vi "frequency_sweep.vi"() -> ()   [LabVIEW 2017]
uses:
  controls/State.ctl
  controls/Data.ctl
  <vilib>/Utility/error.llb/DialogType.ctl
  <vilib>/DAQmx/write.llb/DAQmx Write (Analog DBL 1Chan 1Samp).vi
  <vilib>/DAQmx/create/channels.llb/DAQmx Create Channel (AO-Voltage-Basic).vi
  <vilib>/DAQmx/miscellaneous.llb/DAQmx Fill In Error Info.vi
  <instrlib>/niVNA/niVNA.llb/niVNA Fetch Sweep Measurement (DBL).vi
panel:
  in  "Reference H Field On/Off":bool
  out "DAQ channel Out":tag="DAQ_6363/ao1"
  in  "Averaging Points":i32=4 min=1 max=3201 step=1
  in  "DAQ channel In":tag="DAQ_6363/ao1"
  in  "Exit Button":bool
  in  "IF Bandwidth":dbl(ring)=1000.0 items=["10 Hz"=10.0, "30 Hz"=30.0, "100 Hz"=100.0, "300 Hz"=300.0, "1 KHz"=1000.0, "3 KHz"=3000.0, "10 KHz"=10000.0, "30 KHz"=30000.0]
  in  "Reference H Field (Oe)":dbl=5500.0 min=-6000.0 max=6000.0
  in  "H Field (Oe)":dbl=1000.0 min=-6000.0 max=6000.0
  in  "Save Button":bool
  out "Status":string="Shutting down...Sweeping field to zero..."
  out "Cursor":cluster{"x":dbl, "y":dbl} {"x" format="%.2f"; "y" format="%.5f"}
  out "VNA Name Out":refnum<k15>="VNA_5630"
  out "Error Out":errorcluster
  in  "Error In (no error)":errorcluster
  in  "Format":i32(ring)=1 items=["Log Magnitude (dB)"=0, "Lin Magnitude"=1, "Phase (deg)"=2, "VSWR"=3, "Group Delay"=6]
  out "SpectrumGraph":cluster{"Field":dbl[], "Signal":dbl[]}(graph)
  in  "S-parameter":i32(ring)=1 caption="Measurement" items=["S11", "S21"]
  in  "Start Button":bool
  in  "Stop Button":bool
  in  "Output Power (dBm)":dbl=1.0 min=-25.0 max=5.0 step=0.5
  in  "Number of Points":i32=1000 min=1 max=3201 step=1
  in  "Stop frequency (GHz)":dbl=6.0 caption="Stop H Field (Oe)" min=0.01 max=6.0 format="%#_6f"
  in  "Start frequency (GHz)":dbl=1.0 min=0.01 max=6.0 format="%#_6f"
  in  "VNA Name In":refnum<k15>="VNA_5630"
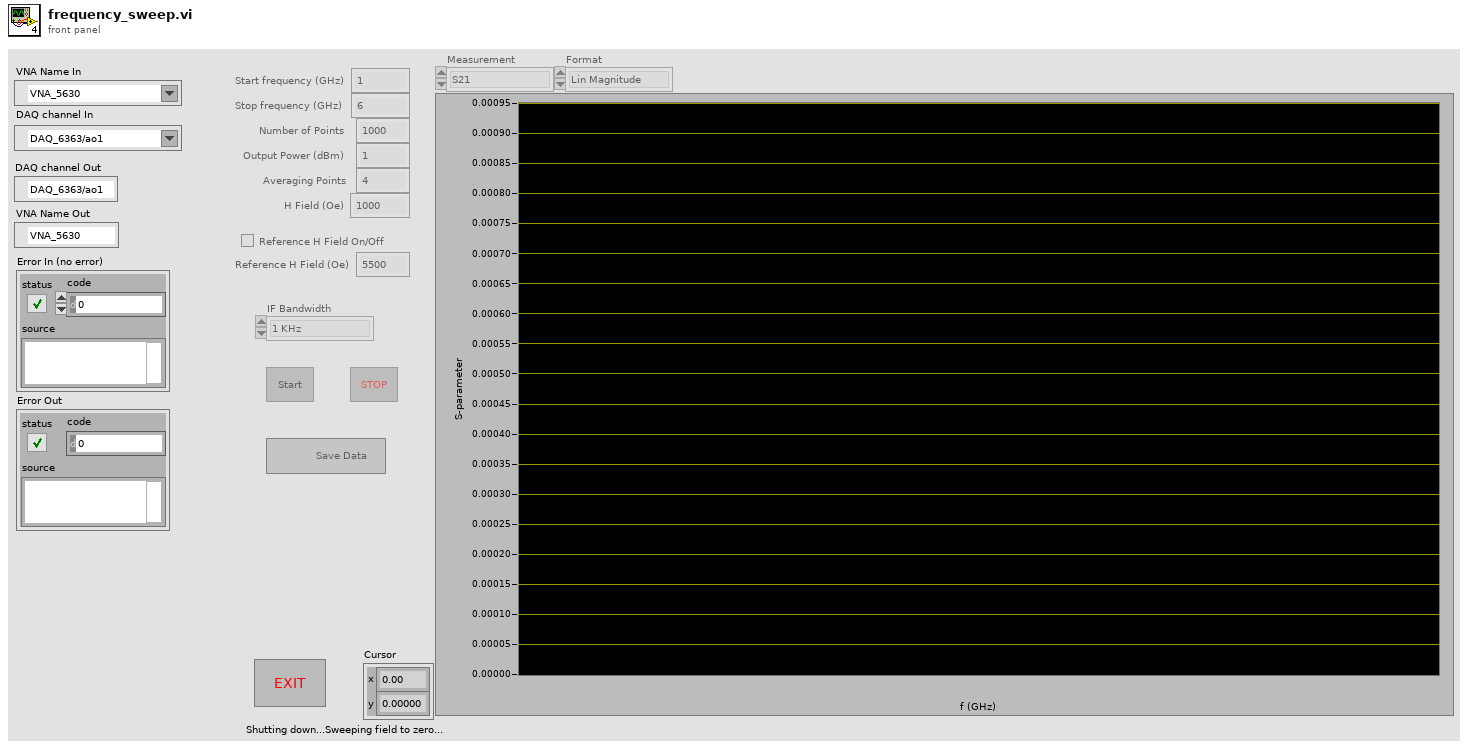
[diagram p1: front panel]
types:
  T1 = typedef "Data.ctl" = cluster{"Frequency":dbl[], "Signal":dbl[], "Ref signal":dbl[]}
  T2 = typedef "State.ctl" = enum16{"Init", "Idle", "Configuring", "Sweeping to ref", "Measuring ref", "Sweeping to H", "Measuring H", "Sweeping down", "Shutdown"}
  T3 = typedef "DialogType.ctl" = u16
  T4 = typedef "LVPoint32TypeDef.ctl" = cluster{"Horizontal":i32, "Vertical":i32}
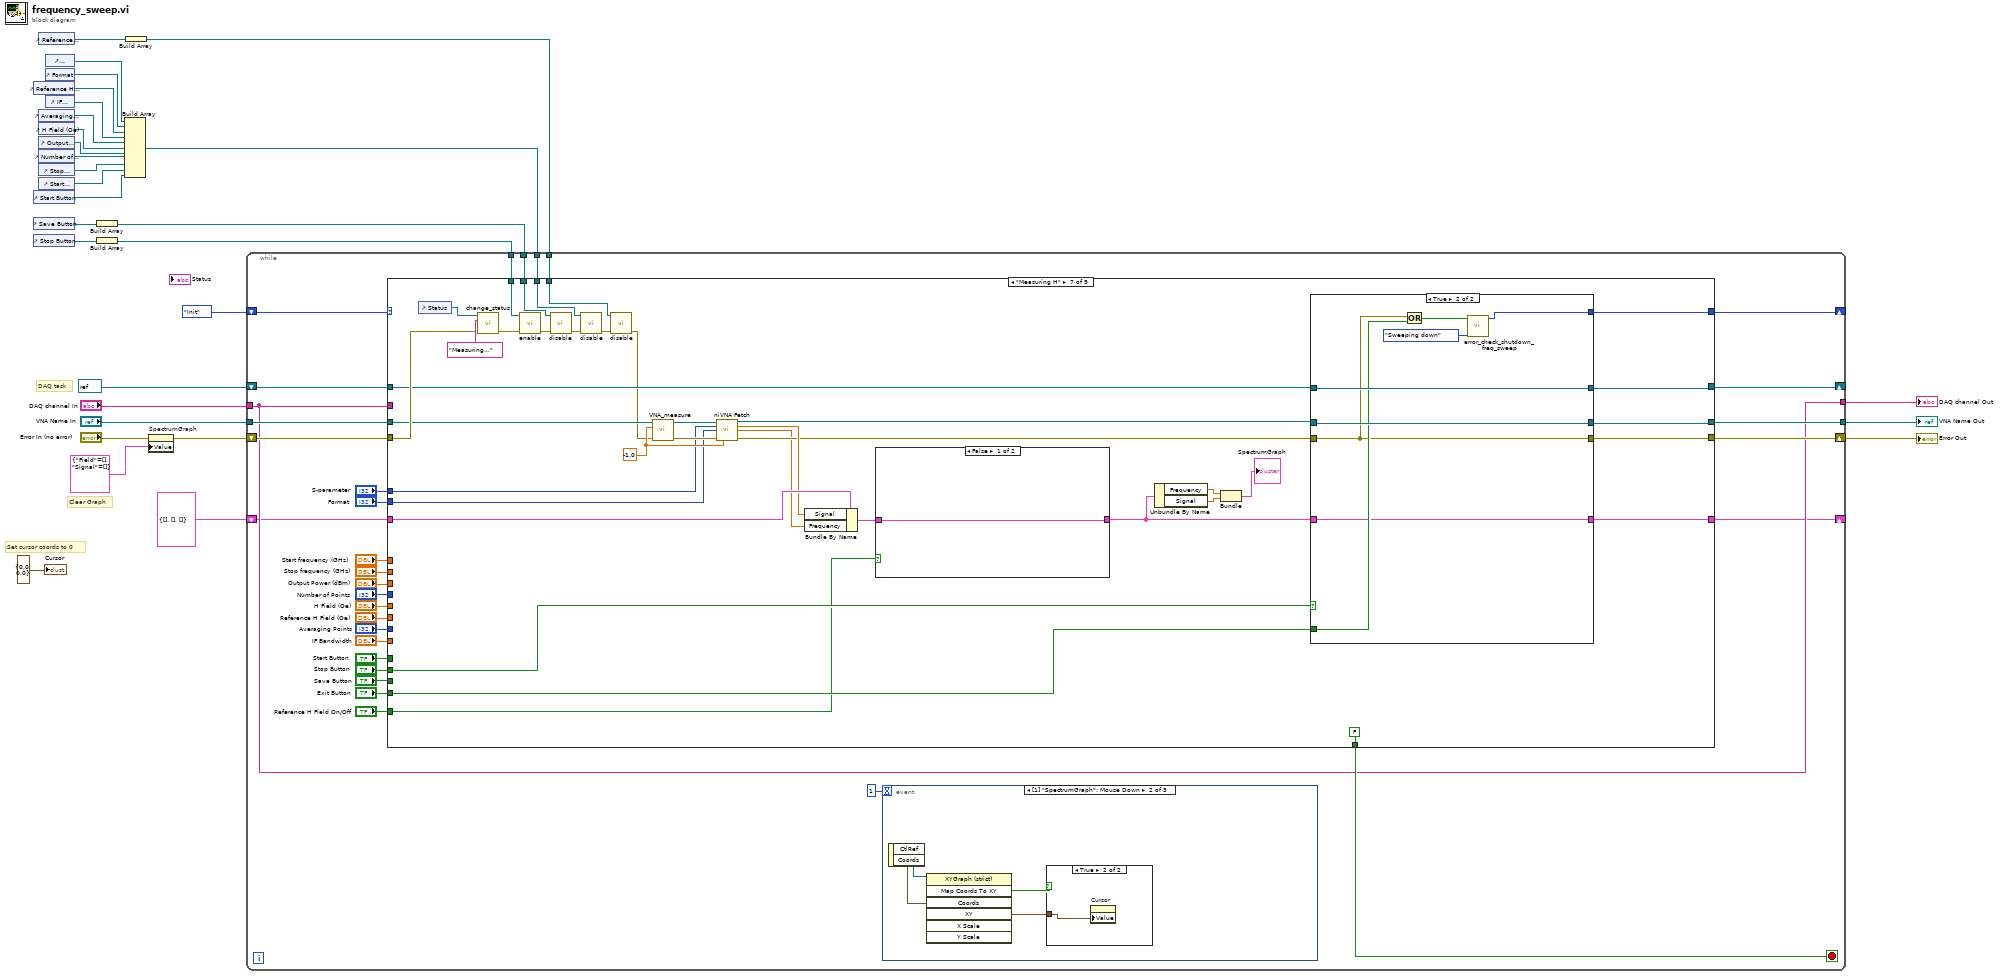
[diagram p0: block diagram]
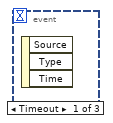
[diagram p2: hidden frame]
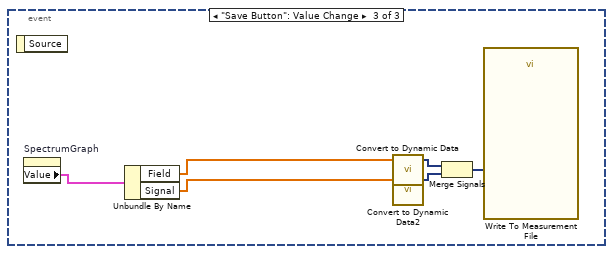
[diagram p4: hidden frame]
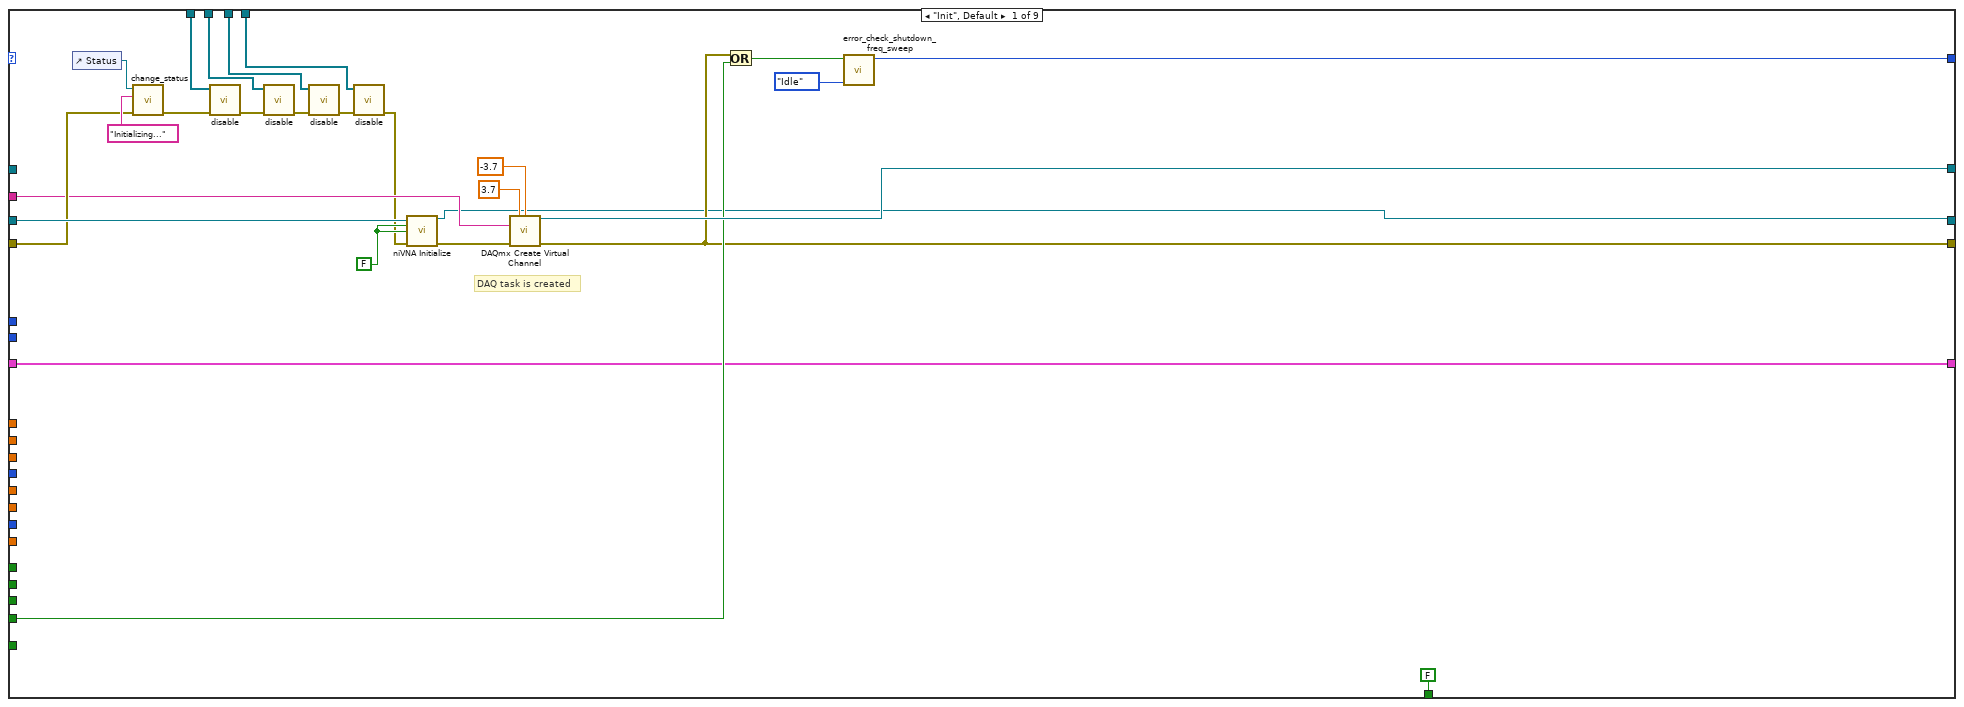
[diagram p5: hidden frame]
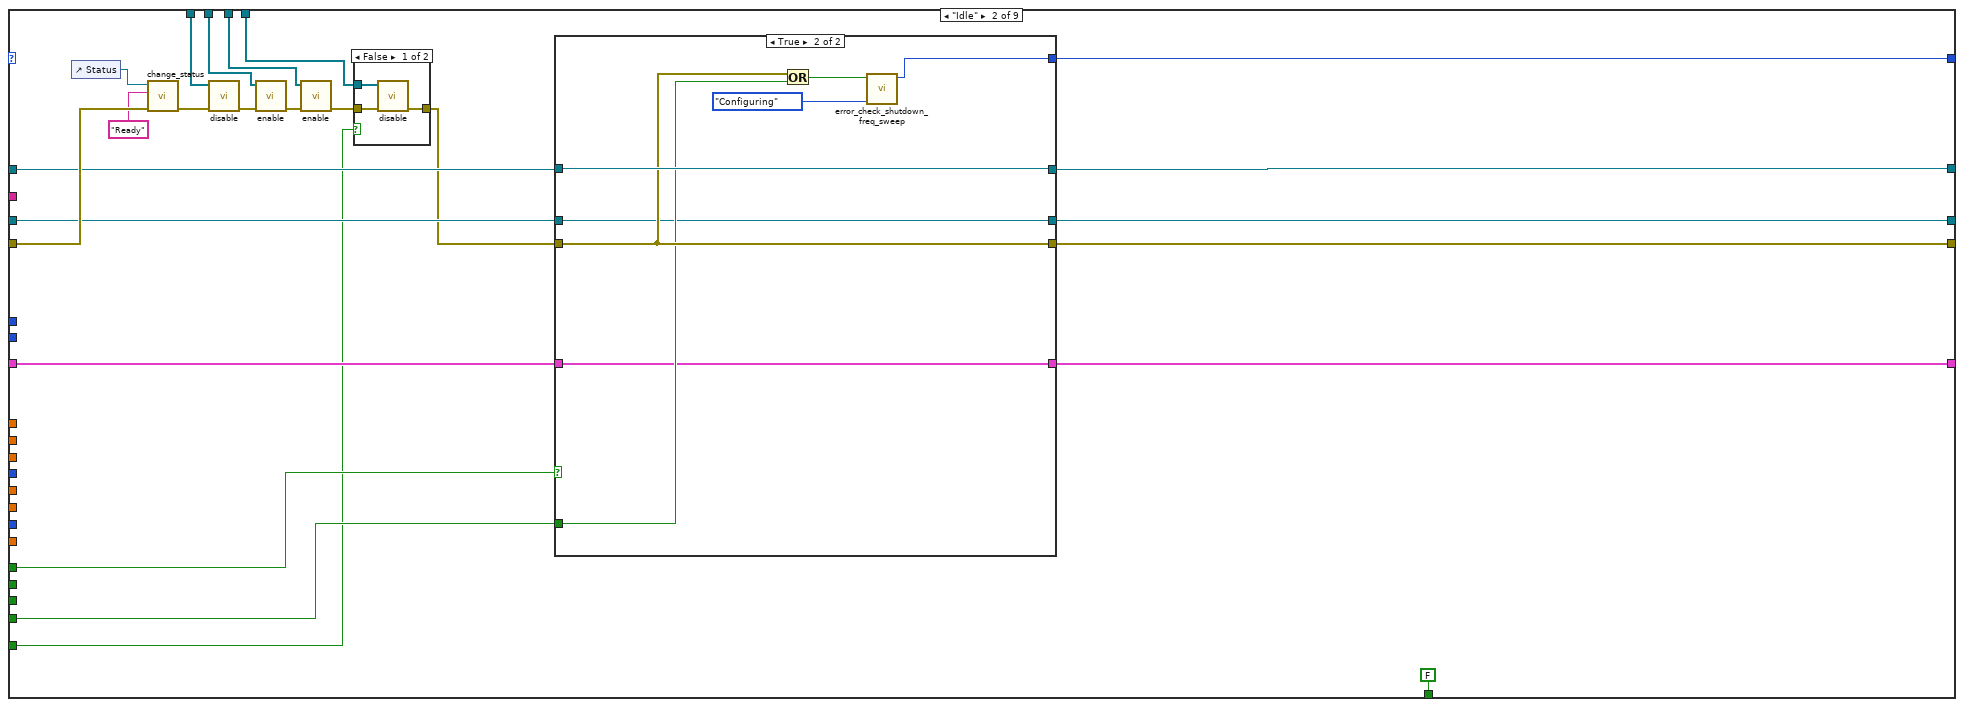
[diagram p6: hidden frame]
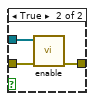
[diagram p7: hidden frame]
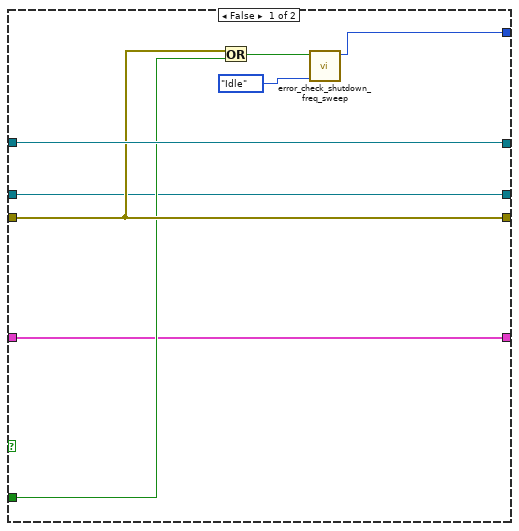
[diagram p8: hidden frame]
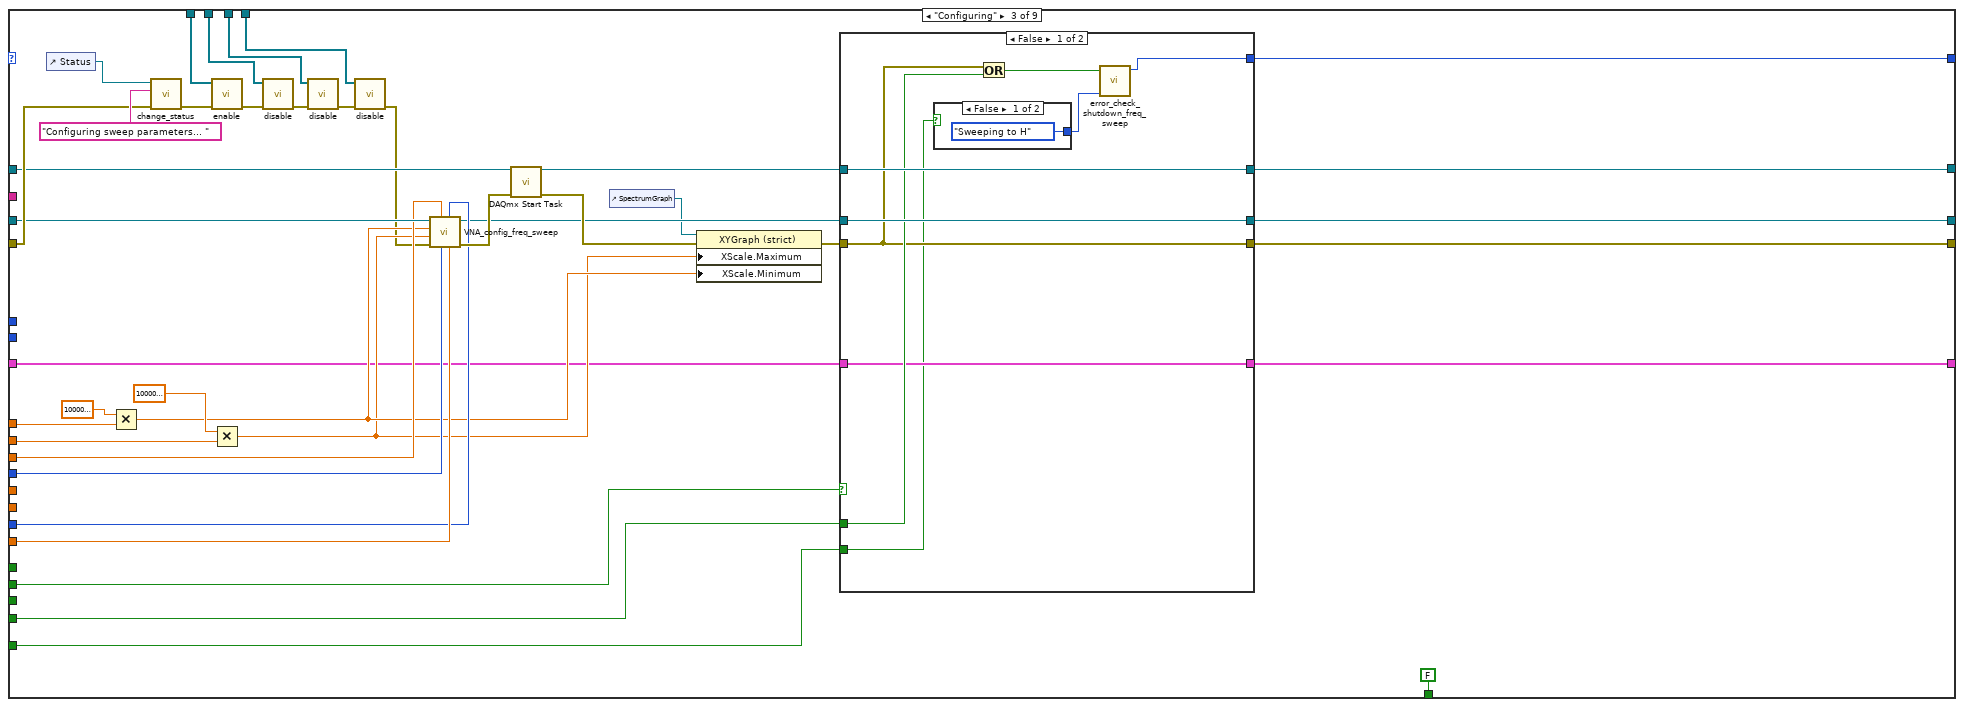
[diagram p9: hidden frame]
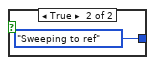
[diagram p10: hidden frame]
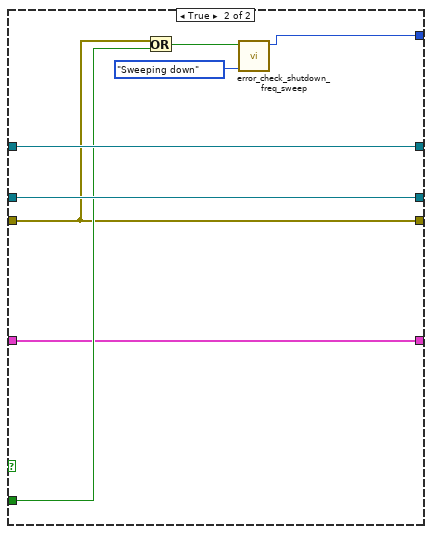
[diagram p11: hidden frame]
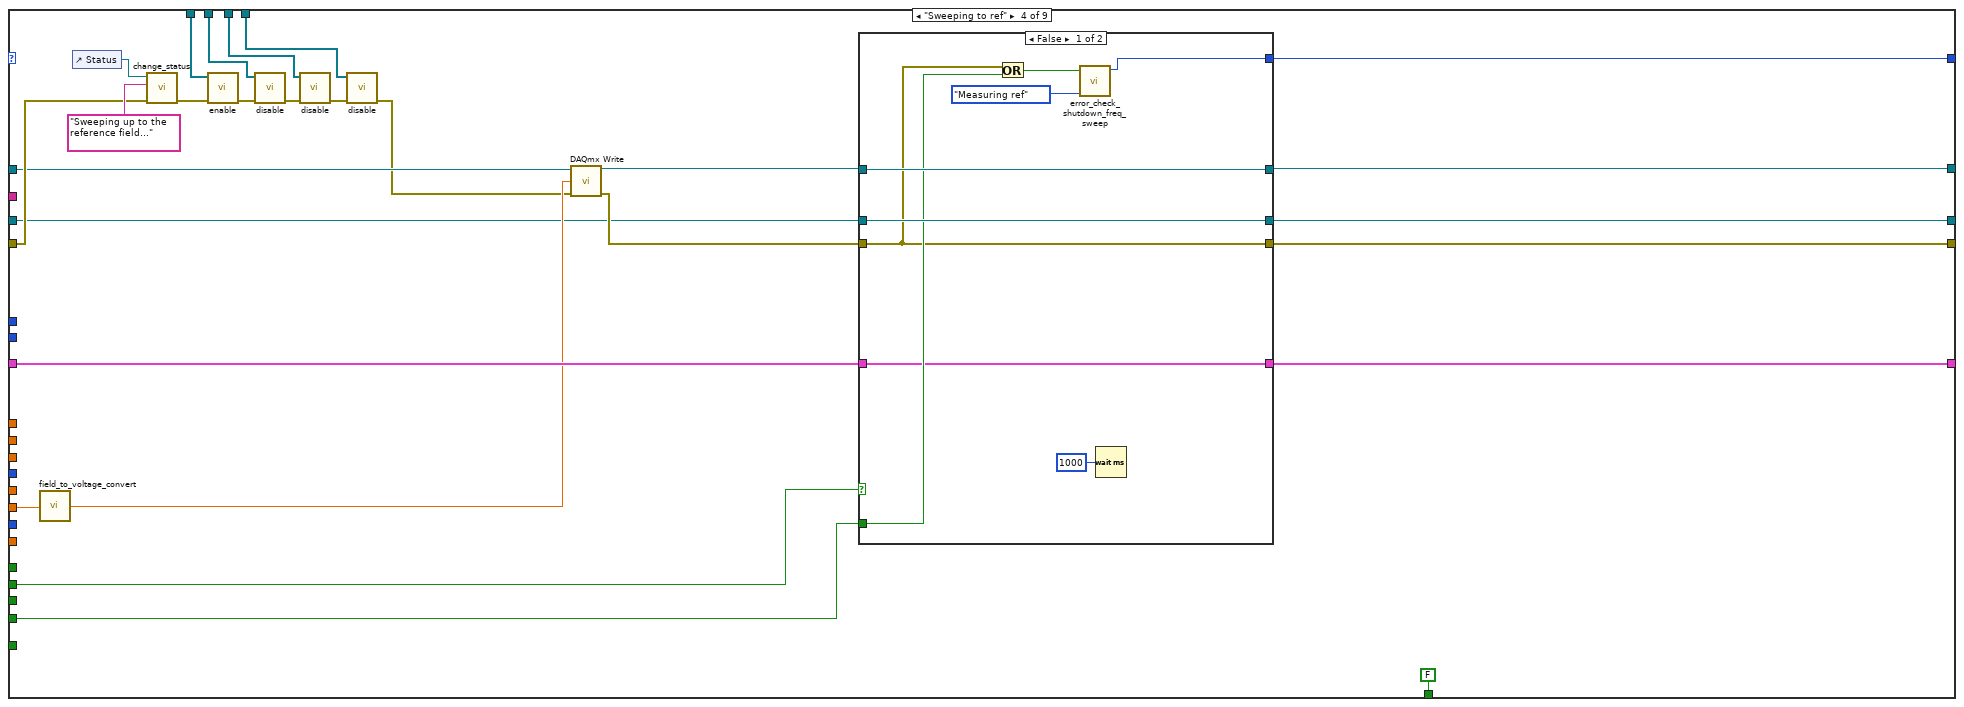
[diagram p12: hidden frame]
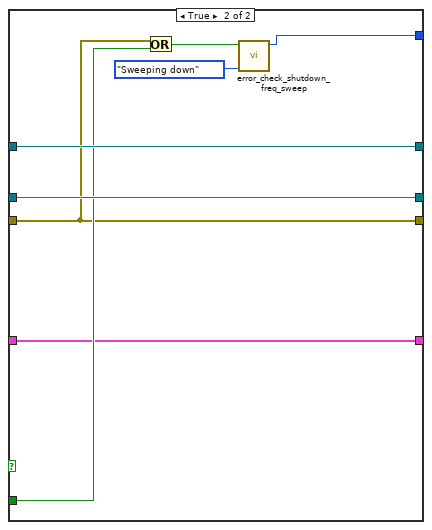
[diagram p13: hidden frame]
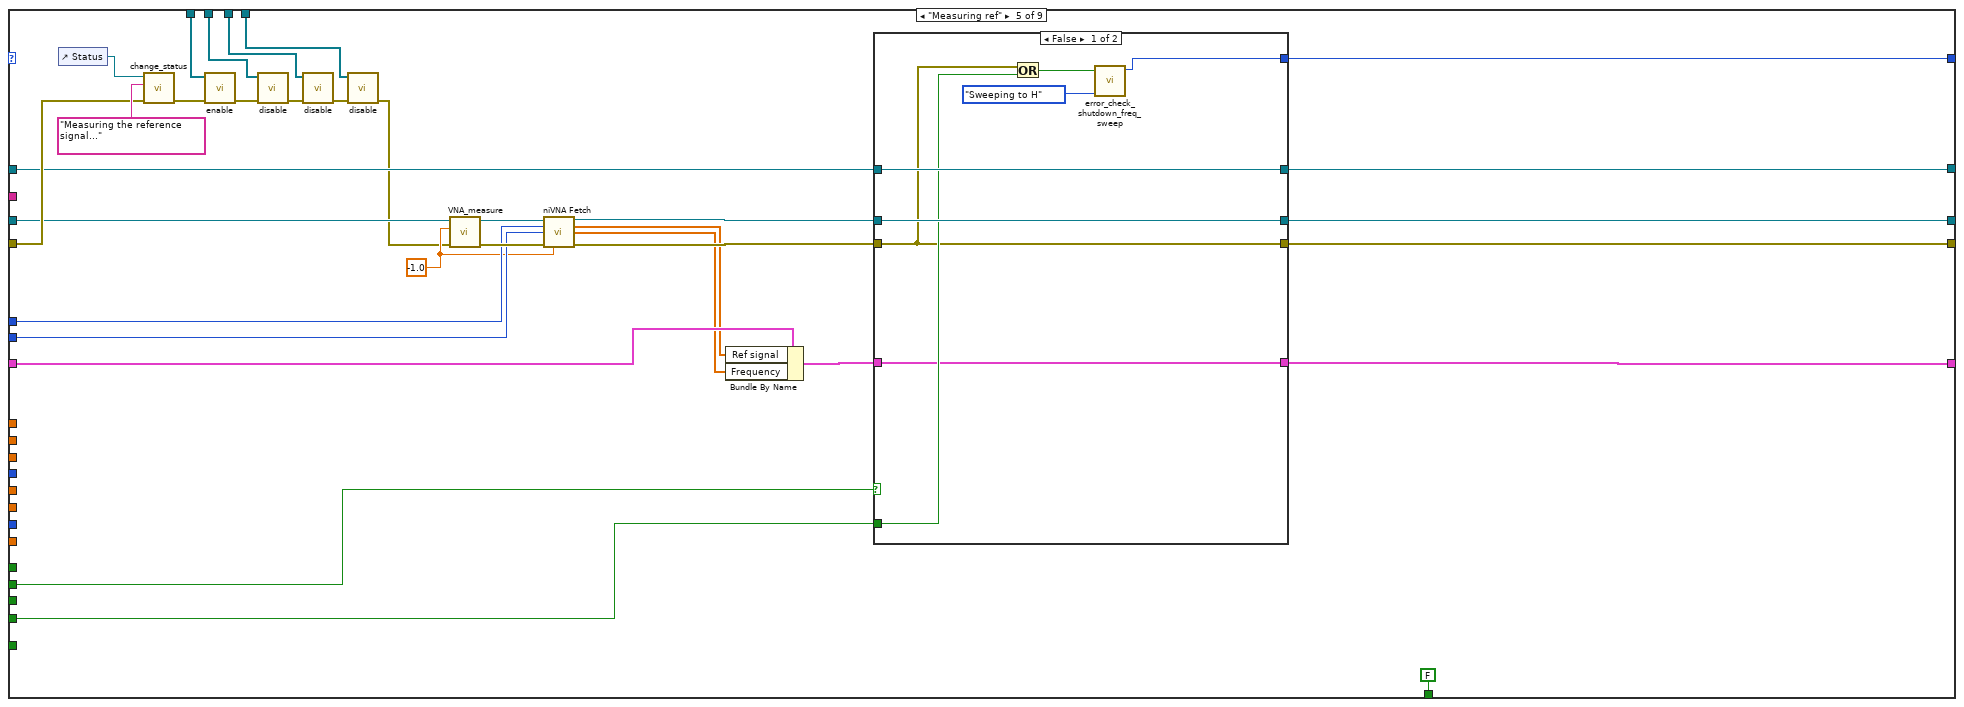
[diagram p14: hidden frame]
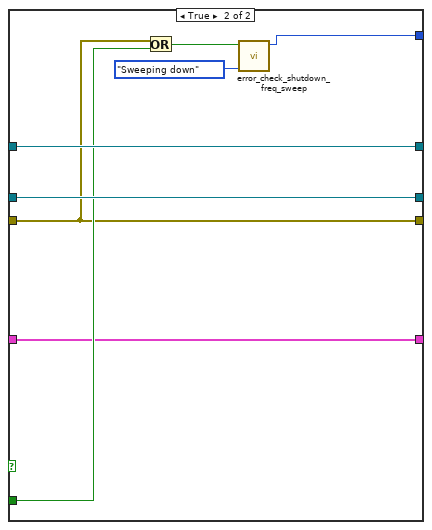
[diagram p15: hidden frame]
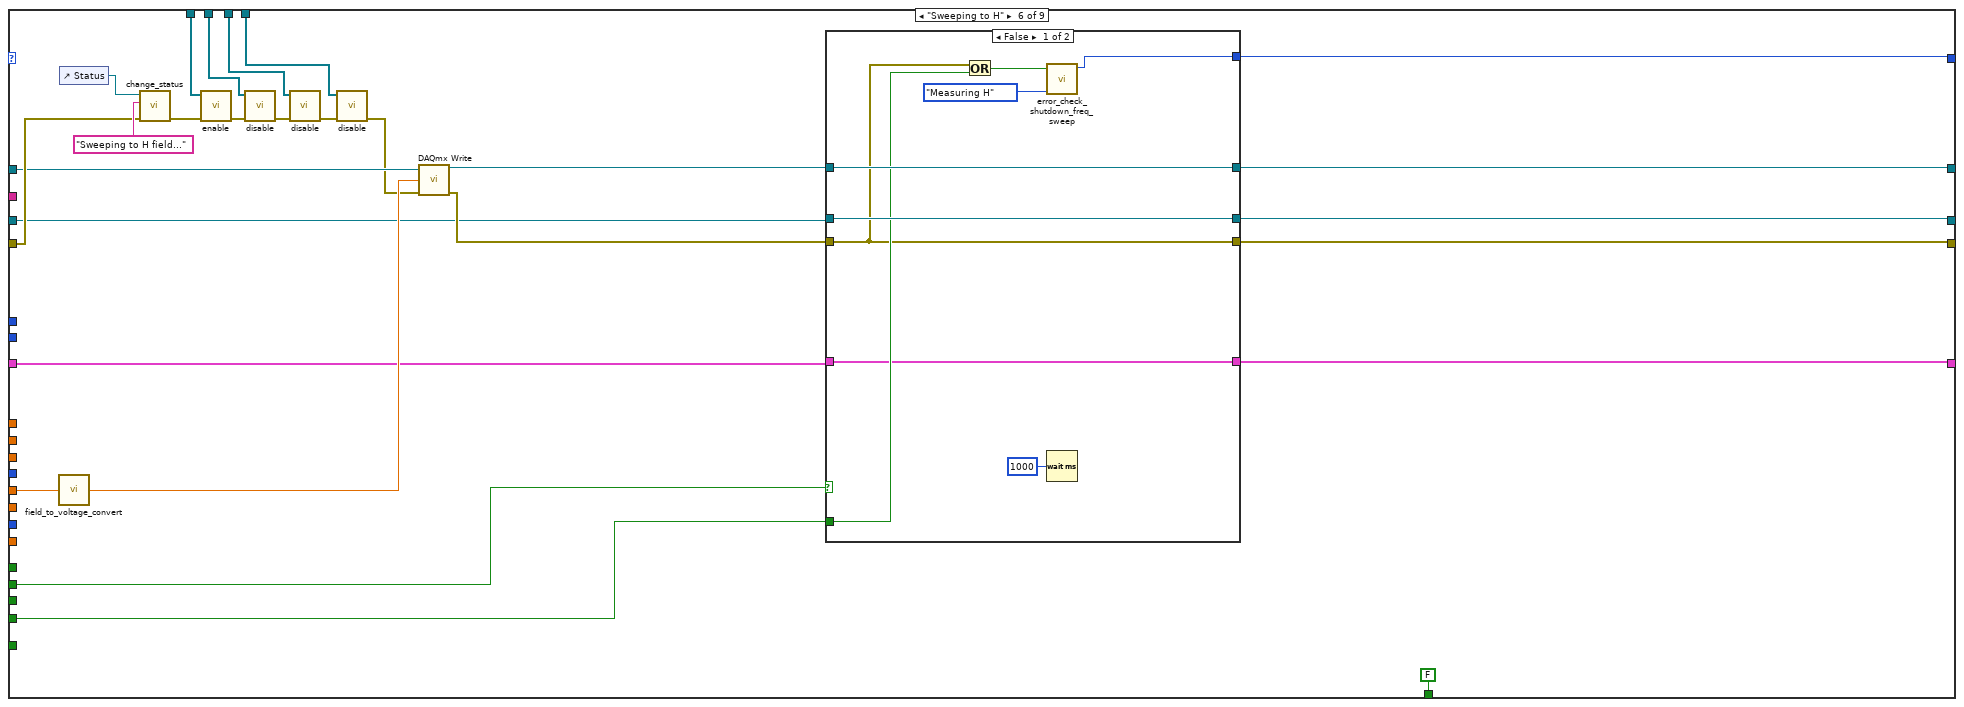
[diagram p16: hidden frame]
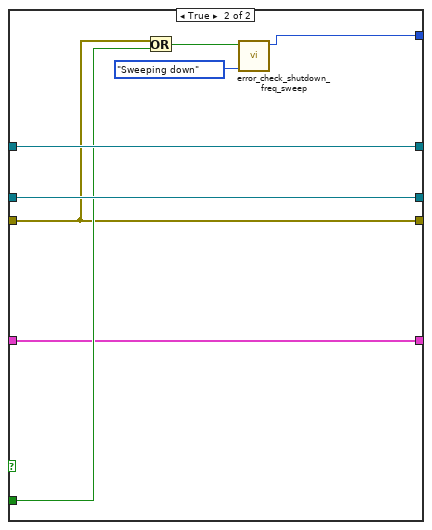
[diagram p17: hidden frame]
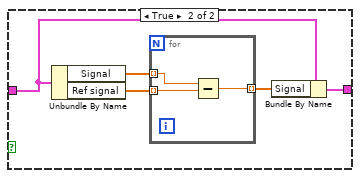
[diagram p18: hidden frame]
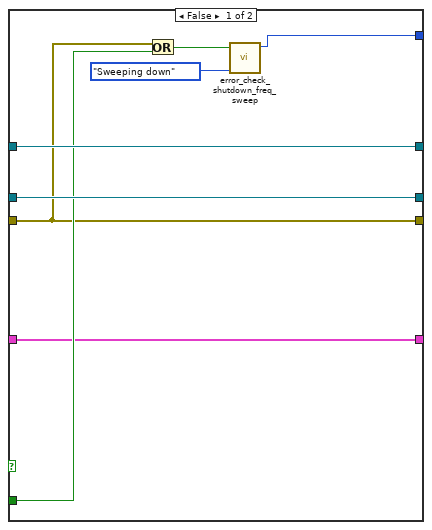
[diagram p19: hidden frame]
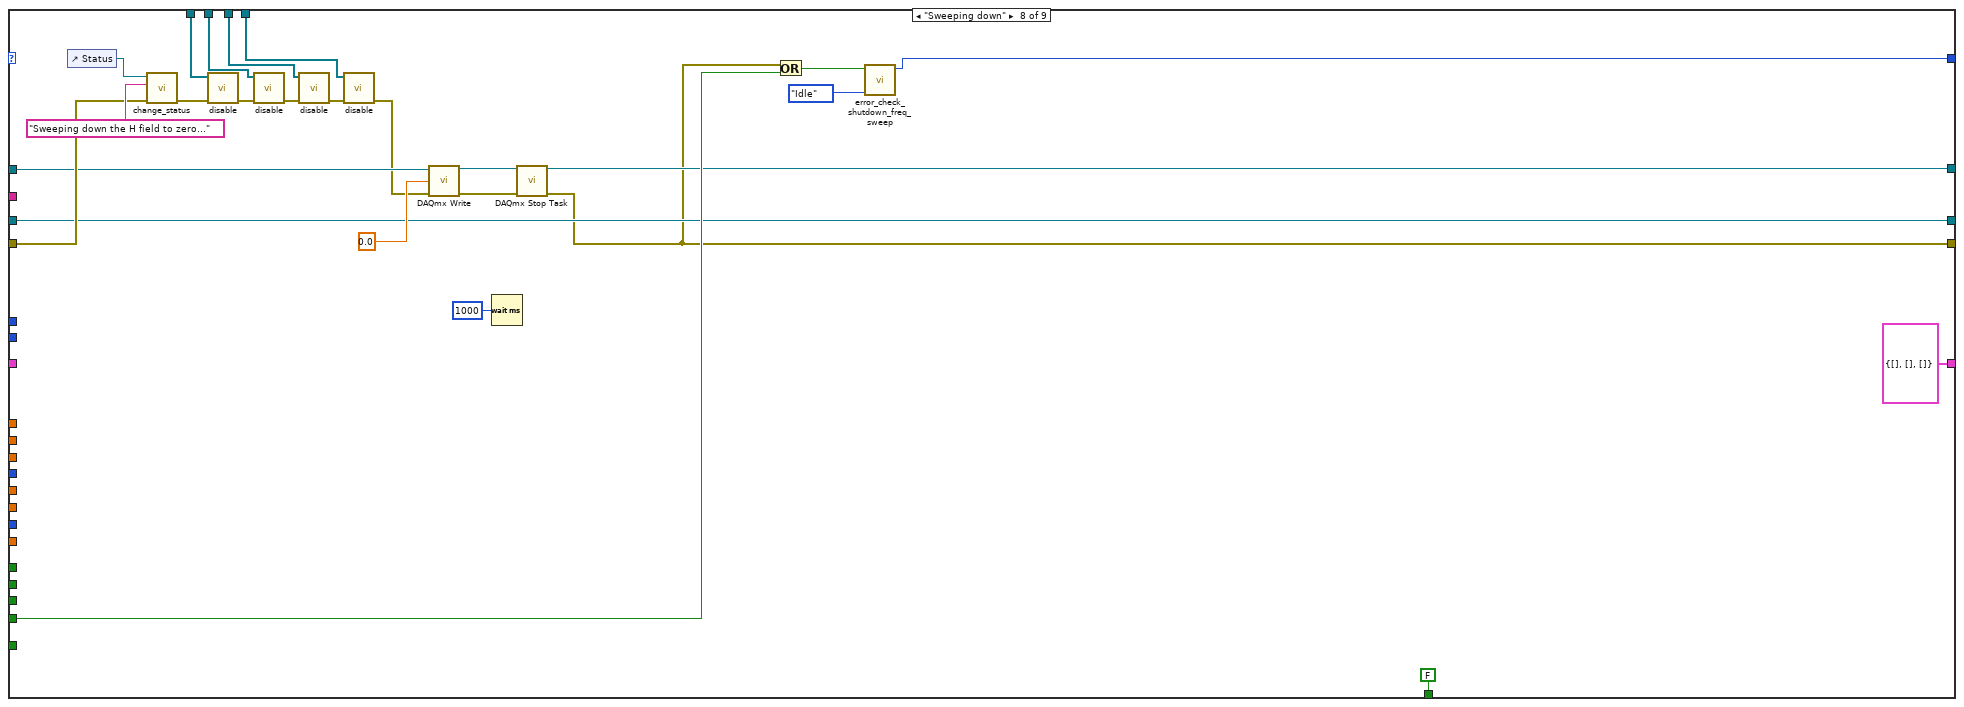
[diagram p20: hidden frame]
diagram:
  # "DAQ task"
  # "Set cursor coords to 0"
  # "Clear Graph"
  n1 = control-ref of="Reference H Field On/Off"() -> (w6:refnum<vi>)
  n2 = control-ref of="Start Button"() -> (w3:refnum<vi>)
  n3 = control-ref of="Save Button"() -> (w17:refnum<vi>)
  n4 = control-ref of="Stop Button"() -> (w23:refnum<vi>)
  n5 = control-ref of="Reference H Field (Oe)"() -> (w5:refnum<vi>)
  n6 = control-ref of="Averaging Points"() -> (w15:refnum<vi>)
  n7 = control-ref of="H Field (Oe)"() -> (w28:refnum<vi>)
  n8 = control-ref of="Output Power (dBm)"() -> (w27:refnum<vi>)
  n9 = control-ref of="Number of Points"() -> (w26:refnum<vi>)
  n10 = control-ref of="Stop frequency (GHz)"() -> (w25:refnum<vi>)
  n11 = control-ref of="Start frequency (GHz)"() -> (w24:refnum<vi>)
  n12 = control-ref of="S-parameter"() -> (w1:refnum<vi>)
  n13 = control-ref of="Format"() -> (w2:refnum<vi>)
  n14 = control-ref of="IF Bandwidth"() -> (w29:refnum<vi>)
  n15 = Build Array(w17) -> (w16:refnum<vi>[])
  n16 = Build Array(w23) -> (w21:refnum<vi>[])
  n17 = Build Array(w1, w2, w6, w29, w15, w28, w27, w26, w25, w24, w3) -> (w22:refnum<vi>[])
  n18 = Build Array(w5) -> (w4:refnum<vi>[])
  n19 = property on="SpectrumGraph" class="XYGraph (strict)"(error in="Error In (no error)", "Value"=cluster{"Field":dbl[], "Signal":dbl[]} {"Field"=[], "Signal"=[]} ("SpectrumGraph")) -> (error out=w10:errorcluster)  [unwired: 1 in, 1 out]
  n20 = while {
    shift-right: [w33] -> _
    shift-left: State."Init" -> [w36]
    tunnel: w22 -> [w62]
    tunnel: w21 -> [w61]
    tunnel: "VNA Name In" -> [w60]
    tunnel: "DAQ channel In" -> [w41]
    shift-right: [w59] -> w14
    shift-left: w10 -> [w58]
    shift-right: [w57] -> _
    shift-left: refnum<k21> refnum ("task in") -> [w56]
    tunnel: w16 -> [w55]
    tunnel: [w43] -> w13
    shift-right: [w37] -> _
    shift-left: T1 {"Frequency"=[], "Signal"=[], "Ref signal"=[]} -> [w38]
    tunnel: [w41] -> w12
    tunnel: w4 -> [w31]
    stop <- w50 stop-if-true
    n21 = case shown="\"Measuring H\"" w36 {
      tunnel: w62 -> [w87 w122 w182 w227 w280 w320 w375 w425 w459]
      tunnel: w61 -> [w100 w124 w181 w229 w282 w323 w377 w423 w461]
      tunnel: w60 -> [w95 w114 w178 w210 w274 w311 w369 w419 w447]
      tunnel: w58 -> [w94 w119 w179 w225 w275 w318 w374 w428 w457]
      tunnel: [w84 w106 w157 w219 w263 w307 w350 w420 State."Shutdown" ("Enum")] -> w33
      tunnel: w41 -> [w90 _ _ _ _ _ _ _ _]
      tunnel: [w83 w115 w154 w223 w260 w304 w353 w412 w435] -> w59
      tunnel: [w89 w112 w156 w221 w262 w306 w351 w414 w453] -> w57
      tunnel: w56 -> [_ w113 w177 w211 w265 w317 w356 w426 w450]
      tunnel: w55 -> [w88 w123 w183 w228 w281 w321 w376 w424 w460]
      tunnel: "Start Button" -> [_ w116 _ _ _ _ _ _ _]
      tunnel: "Stop Button" -> [_ _ w160 w224 w268 w309 w355 _ _]
      tunnel: "Save Button" -> [_ _ _ _ _ _ _ _ _]
      tunnel: "Exit Button" -> [w85 w111 w159 w218 w267 w308 w354 w421 _]
      tunnel: [FALSE FALSE FALSE FALSE FALSE FALSE FALSE FALSE TRUE] -> w50
      tunnel: "Start frequency (GHz)" -> [_ _ w172 _ _ _ _ _ _]
      tunnel: "Stop frequency (GHz)" -> [_ _ w171 _ _ _ _ _ _]
      tunnel: "Output Power (dBm)" -> [_ _ w168 _ _ _ _ _ _]
      tunnel: "Number of Points" -> [_ _ w170 _ _ _ _ _ _]
      tunnel: "H Field (Oe)" -> [_ _ _ _ _ w315 _ _ _]
      tunnel: "Reference H Field (Oe)" -> [_ _ _ w214 _ _ _ _ _]
      tunnel: [w81 w110 w155 w222 w261 w305 w352 w419 w454] -> w43
      tunnel: "Averaging Points" -> [_ _ w167 _ _ _ _ _ _]
      tunnel: w38 -> [w79 w109 w161 w217 w258 w310 w366 _ _]
      tunnel: "IF Bandwidth" -> [_ _ w169 _ _ _ _ _ _]
      tunnel: [w79 w107 w153 w215 w256 w303 w359 T1 {"Frequency"=[], "Signal"=[], "Ref signal"=[]} T1 {"Frequency"=[], "Signal"=[], "Ref signal"=[]}] -> w37
      tunnel: "S-parameter" -> [_ _ _ _ w271 _ w368 _ _]
      tunnel: "Format" -> [_ _ _ _ w270 _ w367 _ _]
      tunnel: "Reference H Field On/Off" -> [_ w104 w158 _ _ _ w347 _ _]
      tunnel: w31 -> [w75 w101 w148 w206 w251 w300 w344 w407 w440]
      frame "Init", Default {
        w96 = FALSE ("id query")
        # "DAQ task is created"
        n22 = control-ref of="Status"() -> (w98:refnum<vi>)
        n23 = call "change_status.vi"("error in (no error)"=w94, "String"="Initializing...", "String in"=w98) -> ("error out"=w99:errorcluster)  [unwired: 8 in]
        n24 = call "disable.vi"("error in (no error)"=w99, "Array"=w100) -> ("error out"=w77:errorcluster)  [unwired: 9 in]
        n25 = call "disable.vi"("error in (no error)"=w77, "Array"=w88) -> ("error out"=w86:errorcluster)  [unwired: 9 in]
        n26 = call "disable.vi"("error in (no error)"=w86, "Array"=w87) -> ("error out"=w76:errorcluster)  [unwired: 9 in]
        n27 = call "disable.vi"("error in (no error)"=w76, "Array"=w75) -> ("error out"=w74:errorcluster)  [unwired: 9 in]
        n28 = call <instrlib>:"niVNA Initialize.vi"("resource name"=w95, "id query"=w96, "reset"=w96, "error in"=w74) -> ("instrument handle"=w81:refnum<k15>, "error out"=w93:errorcluster)  [unwired: 10 in]
        n29 = call-poly <vilib>:"DAQmx Create Virtual Channel.vi"("maximum value"=3.7, "minimum value"=-3.7, "physical channels"=w90, "error in"=w93) -> ("task out"=w89:refnum<k21>, "error out"=w83:errorcluster)  [unwired: 10 in]
        n30 = Or(x=w83, y=w85) -> (x .or. y?=w82:bool)
        n31 = call "error_check_shutdown_freq_sweep.vi"(8:State."Idle", "Boolean"=w82) -> (3:w84:T2)  [unwired: 9 in]
      }
      frame "Idle" {
        n32 = control-ref of="Status"() -> (w118:refnum<vi>)
        n33 = call "change_status.vi"("error in (no error)"=w119, "String"="Ready", "String in"=w118) -> ("error out"=w120:errorcluster)  [unwired: 8 in]
        n34 = call "disable.vi"("error in (no error)"=w120, "Array"=w124) -> ("error out"=w105:errorcluster)  [unwired: 9 in]
        n35 = call "enable.vi"("error in (no error)"=w105, "Array"=w123) -> ("error out"=w121:errorcluster)  [unwired: 9 in]
        n36 = call "enable.vi"("error in (no error)"=w121, "Array"=w122) -> ("error out"=w103:errorcluster)  [unwired: 9 in]
        n37 = case shown="False" w104 {
          tunnel: w103 -> [w127 w130]
          tunnel: [w125 w129] -> w102
          tunnel: w101 -> [w126 w128]
          frame False {
            n38 = call "disable.vi"("error in (no error)"=w127, "Array"=w126) -> ("error out"=w125:errorcluster)  [unwired: 9 in]
          }
          frame True {
            n39 = call "enable.vi"("error in (no error)"=w130, "Array"=w128) -> ("error out"=w129:errorcluster)  [unwired: 9 in]
          }
        }
        n40 = case shown="True" w116 {
          tunnel: w102 -> [w137 w145]
          tunnel: [w137 w145] -> w115
          tunnel: w114 -> [w135 w143]
          tunnel: w113 -> [w138 w146]
          tunnel: [w138 w146] -> w112
          tunnel: [w131 w140] -> w106
          tunnel: w111 -> [w136 w144]
          tunnel: [w135 w143] -> w110
          tunnel: w109 -> [w134 w142]
          tunnel: [w134 w142] -> w107
          frame False {
            n41 = Or(x=w137, y=w136) -> (x .or. y?=w133:bool)
            n42 = call "error_check_shutdown_freq_sweep.vi"(8:State."Idle", "Boolean"=w133) -> (3:w131:T2)  [unwired: 9 in]
          }
          frame True {
            n43 = Or(x=w145, y=w144) -> (x .or. y?=w141:bool)
            n44 = call "error_check_shutdown_freq_sweep.vi"(8:State."Configuring", "Boolean"=w141) -> (3:w140:T2)  [unwired: 9 in]
          }
        }
      }
      frame "Configuring" {
        n45 = control-ref of="Status"() -> (w180:refnum<vi>)
        n46 = Multiply(x=1000000000.0, y=w172) -> (x*y=w166:dbl)
        n47 = call "change_status.vi"("error in (no error)"=w179, "String"="Configuring sweep parameters... ", "String in"=w180) -> ("error out"=w185:errorcluster)  [unwired: 8 in]
        n48 = call "enable.vi"("error in (no error)"=w185, "Array"=w181) -> ("error out"=w150:errorcluster)  [unwired: 9 in]
        n49 = Multiply(x=1000000000.0, y=w171) -> (x*y=w165:dbl)
        n50 = call "disable.vi"("error in (no error)"=w150, "Array"=w183) -> ("error out"=w186:errorcluster)  [unwired: 9 in]
        n51 = call "disable.vi"("error in (no error)"=w186, "Array"=w182) -> ("error out"=w149:errorcluster)  [unwired: 9 in]
        n52 = call "disable.vi"("error in (no error)"=w149, "Array"=w148) -> ("error out"=w147:errorcluster)  [unwired: 9 in]
        n53 = call "VNA_config_freq_sweep.vi"("IF Bandwidth"=w169, "Averaging"=w167, "Number of Points"=w170, "Output Power"=w168, "error in (no error)"=w147, "Stop Frequency"=w165, "Start Frequency"=w166, "Resource Name In"=w178) -> ("error out"=w176:errorcluster, "Resource Name Out"=w162:refnum<k15>)  [unwired: 2 in]
        n54 = call <vilib>:"DAQmx Start Task.vi"("task/channels in"=w177, "error in"=w176) -> ("task out"=w164:refnum<k21>, "error out"=w175:errorcluster)  [unwired: 12 in]
        n55 = control-ref of="SpectrumGraph"() -> (w151:refnum<vi>)
        n56 = property on="Property Node" class="XYGraph (strict)"(reference=w151, error in=w175, "XScale.Maximum"=w165, "XScale.Minimum"=w166) -> (error out=w163:errorcluster)  [unwired: 1 out]
        n57 = case shown="False" w160 {
          tunnel: w163 -> [w192 w202]
          tunnel: w164 -> [w195 w204]
          tunnel: w162 -> [w194 w205]
          tunnel: [w192 w202] -> w154
          tunnel: [w194 w205] -> w155
          tunnel: [w195 w204] -> w156
          tunnel: [w188 w199] -> w157
          tunnel: w159 -> [w193 w203]
          tunnel: w161 -> [w191 w201]
          tunnel: [w191 w201] -> w153
          tunnel: w158 -> [w187 _]
          frame False {
            n58 = case shown="False" w187 {
              tunnel: [State."Sweeping to H" State."Sweeping to ref"] -> w189
              frame False {
              }
              frame True {
              }
            }
            n59 = Or(x=w192, y=w193) -> (x .or. y?=w190:bool)
            n60 = call "error_check_shutdown_freq_sweep.vi"(8:w189, "Boolean"=w190) -> (3:w188:T2)  [unwired: 9 in]
          }
          frame True {
            n61 = Or(x=w202, y=w203) -> (x .or. y?=w200:bool)
            n62 = call "error_check_shutdown_freq_sweep.vi"(8:State."Sweeping down", "Boolean"=w200) -> (3:w199:T2)  [unwired: 9 in]
          }
        }
      }
      frame "Sweeping to ref" {
        n63 = call "field_to_voltage_convert.vi"("Start H Field (Oe)"=w214) -> ("Numeric"=w213:dbl)
        n64 = control-ref of="Status"() -> (w226:refnum<vi>)
        n65 = call "change_status.vi"("error in (no error)"=w225, "String"="Sweeping up to the reference field...", "String in"=w226) -> ("error out"=w231:errorcluster)  [unwired: 8 in]
        n66 = call "enable.vi"("error in (no error)"=w231, "Array"=w229) -> ("error out"=w209:errorcluster)  [unwired: 9 in]
        n67 = call "disable.vi"("error in (no error)"=w209, "Array"=w228) -> ("error out"=w230:errorcluster)  [unwired: 9 in]
        n68 = call "disable.vi"("error in (no error)"=w230, "Array"=w227) -> ("error out"=w208:errorcluster)  [unwired: 9 in]
        n69 = call "disable.vi"("error in (no error)"=w208, "Array"=w206) -> ("error out"=w207:errorcluster)  [unwired: 9 in]
        n70 = call-poly <vilib>:"DAQmx Write.vi"("task/channels in"=w211, "data"=w213, "error in"=w207) -> ("task out"=w220:refnum<k21>, "error out"=w212:errorcluster)  [unwired: 10 in, 1 out]
        n71 = case shown="False" w224 {
          tunnel: w212 -> [w238 w246]
          tunnel: w220 -> [w241 w248]
          tunnel: w210 -> [w240 w249]
          tunnel: [w238 w246] -> w223
          tunnel: [w240 w249] -> w222
          tunnel: [w241 w248] -> w221
          tunnel: [w233 w243] -> w219
          tunnel: w218 -> [w239 w247]
          tunnel: w217 -> [w236 w245]
          tunnel: [w236 w245] -> w215
          frame False {
            n72 = Or(x=w238, y=w239) -> (x .or. y?=w235:bool)
            n73 = call "error_check_shutdown_freq_sweep.vi"(8:State."Measuring ref", "Boolean"=w235) -> (3:w233:T2)  [unwired: 9 in]
            n74 = Wait (ms)(milliseconds to wait=u32 1000) -> ()  [unwired: 1 out]
          }
          frame True {
            n75 = Or(x=w246, y=w247) -> (x .or. y?=w244:bool)
            n76 = call "error_check_shutdown_freq_sweep.vi"(8:State."Sweeping down", "Boolean"=w244) -> (3:w243:T2)  [unwired: 9 in]
          }
        }
      }
      frame "Measuring ref" {
        w269 = -1.0 ("timeout")
        n77 = control-ref of="Status"() -> (w276:refnum<vi>)
        n78 = call "change_status.vi"("error in (no error)"=w275, "String"="Measuring the reference signal...", "String in"=w276) -> ("error out"=w279:errorcluster)  [unwired: 8 in]
        n79 = call "enable.vi"("error in (no error)"=w279, "Array"=w282) -> ("error out"=w253:errorcluster)  [unwired: 9 in]
        n80 = call "disable.vi"("error in (no error)"=w253, "Array"=w281) -> ("error out"=w278:errorcluster)  [unwired: 9 in]
        n81 = call "disable.vi"("error in (no error)"=w278, "Array"=w280) -> ("error out"=w252:errorcluster)  [unwired: 9 in]
        n82 = call "disable.vi"("error in (no error)"=w252, "Array"=w251) -> ("error out"=w250:errorcluster)  [unwired: 9 in]
        n83 = call "VNA_measure.vi"("error in (no error)"=w250, "timeout"=w269, "Resource Name In"=w274) -> ("error out"=w272:errorcluster, "Resource Name Out"=w273:refnum<k15>)  [unwired: 7 in]
        n84 = call-poly <instrlib>:"niVNA Fetch.vi"("instrument handle"=w273, "measurement"=w271, "format"=w270, "error in"=w272, "timeout"=w269) -> ("instrument handle out"=w264:refnum<k15>, "data"=w255:dbl[], "scale points"=w254:dbl[], "error out"=w266:errorcluster)  [unwired: 7 in]
        n85 = Bundle By Name(cluster=w258, "Ref signal"=w255, "Frequency"=w254) -> (w257:T1)
        n86 = case shown="False" w268 {
          tunnel: w266 -> [w287 w295]
          tunnel: w265 -> [w290 w297]
          tunnel: w264 -> [w289 w298]
          tunnel: [w287 w295] -> w260
          tunnel: [w289 w298] -> w261
          tunnel: [w290 w297] -> w262
          tunnel: [w284 w293] -> w263
          tunnel: w267 -> [w288 w296]
          tunnel: [w283 w291] -> w256
          tunnel: w257 -> [w283 w291]
          frame False {
            n87 = Or(x=w287, y=w288) -> (x .or. y?=w286:bool)
            n88 = call "error_check_shutdown_freq_sweep.vi"(8:State."Sweeping to H", "Boolean"=w286) -> (3:w284:T2)  [unwired: 9 in]
          }
          frame True {
            n89 = Or(x=w295, y=w296) -> (x .or. y?=w294:bool)
            n90 = call "error_check_shutdown_freq_sweep.vi"(8:State."Sweeping down", "Boolean"=w294) -> (3:w293:T2)  [unwired: 9 in]
          }
        }
      }
      frame "Sweeping to H" {
        n91 = call "field_to_voltage_convert.vi"("Start H Field (Oe)"=w315) -> ("Numeric"=w314:dbl)
        n92 = control-ref of="Status"() -> (w319:refnum<vi>)
        n93 = call "change_status.vi"("error in (no error)"=w318, "String"="Sweeping to H field...", "String in"=w319) -> ("error out"=w324:errorcluster)  [unwired: 8 in]
        n94 = call "enable.vi"("error in (no error)"=w324, "Array"=w323) -> ("error out"=w302:errorcluster)  [unwired: 9 in]
        n95 = call "disable.vi"("error in (no error)"=w302, "Array"=w321) -> ("error out"=w325:errorcluster)  [unwired: 9 in]
        n96 = call "disable.vi"("error in (no error)"=w325, "Array"=w320) -> ("error out"=w301:errorcluster)  [unwired: 9 in]
        n97 = call "disable.vi"("error in (no error)"=w301, "Array"=w300) -> ("error out"=w299:errorcluster)  [unwired: 9 in]
        n98 = call-poly <vilib>:"DAQmx Write.vi"("task/channels in"=w317, "data"=w314, "error in"=w299) -> ("task out"=w312:refnum<k21>, "error out"=w313:errorcluster)  [unwired: 10 in, 1 out]
        n99 = case shown="False" w309 {
          tunnel: w313 -> [w331 w339]
          tunnel: w312 -> [w334 w341]
          tunnel: w311 -> [w333 w342]
          tunnel: [w331 w339] -> w304
          tunnel: [w333 w342] -> w305
          tunnel: [w334 w341] -> w306
          tunnel: [w327 w336] -> w307
          tunnel: w308 -> [w332 w340]
          tunnel: w310 -> [w330 w338]
          tunnel: [w330 w338] -> w303
          frame False {
            n100 = Or(x=w331, y=w332) -> (x .or. y?=w329:bool)
            n101 = call "error_check_shutdown_freq_sweep.vi"(8:State."Measuring H", "Boolean"=w329) -> (3:w327:T2)  [unwired: 9 in]
            n102 = Wait (ms)(milliseconds to wait=u32 1000) -> ()  [unwired: 1 out]
          }
          frame True {
            n103 = Or(x=w339, y=w340) -> (x .or. y?=w337:bool)
            n104 = call "error_check_shutdown_freq_sweep.vi"(8:State."Sweeping down", "Boolean"=w337) -> (3:w336:T2)  [unwired: 9 in]
          }
        }
      }
      frame "Measuring H" {
        w370 = -1.0 ("timeout")
        n105 = control-ref of="Status"() -> (w373:refnum<vi>)
        n106 = call "change_status.vi"("error in (no error)"=w374, "String"="Measuring...", "String in"=w373) -> ("error out"=w380:errorcluster)  [unwired: 8 in]
        n107 = call "enable.vi"("error in (no error)"=w380, "Array"=w377) -> ("error out"=w346:errorcluster)  [unwired: 9 in]
        n108 = call "disable.vi"("error in (no error)"=w346, "Array"=w376) -> ("error out"=w379:errorcluster)  [unwired: 9 in]
        n109 = call "disable.vi"("error in (no error)"=w379, "Array"=w375) -> ("error out"=w343:errorcluster)  [unwired: 9 in]
        n110 = call "disable.vi"("error in (no error)"=w343, "Array"=w344) -> ("error out"=w345:errorcluster)  [unwired: 9 in]
        n111 = call "VNA_measure.vi"("error in (no error)"=w345, "timeout"=w370, "Resource Name In"=w369) -> ("error out"=w371:errorcluster, "Resource Name Out"=w372:refnum<k15>)  [unwired: 7 in]
        n112 = call-poly <instrlib>:"niVNA Fetch.vi"("instrument handle"=w372, "measurement"=w368, "format"=w367, "error in"=w371, "timeout"=w370) -> ("instrument handle out"=w357:refnum<k15>, "data"=w365:dbl[], "scale points"=w348:dbl[], "error out"=w358:errorcluster)  [unwired: 7 in]
        n113 = Bundle By Name(cluster=w366, "Signal"=w365, "Frequency"=w348) -> (w364:T1)
        n114 = case shown="False" w347 {
          tunnel: w364 -> [w381 w384]
          tunnel: [w381 w382] -> w360
          frame False {
          }
          frame True {
            n115 = Unbundle By Name(w384) -> ("Signal"=w386:dbl[], "Ref signal"=w385:dbl[])
            n116 = for {
              tunnel: w386 -> [w389] mode=indexing
              tunnel: w385 -> [w388] mode=indexing
              tunnel: [w387] -> w383 mode=indexing
              n117 = Subtract(x=w389, y=w388) -> (x-y=w387:dbl)
            }
            n118 = Bundle By Name(cluster=w384, "Signal"=w383) -> (w382:T1)
          }
        }
        n119 = Unbundle By Name(w360) -> ("Frequency"=w363:dbl[], "Signal"=w362:dbl[])
        n120 = Bundle("Frequency"=w363, "Signal"=w362) -> (→"SpectrumGraph":cluster{"Frequency":dbl[], "Signal":dbl[]})  [unwired: 1 in]
        n121 = case shown="True" w355 {
          tunnel: w358 -> [w394 w402]
          tunnel: w356 -> [w397 w404]
          tunnel: w357 -> [w396 w405]
          tunnel: [w394 w402] -> w353
          tunnel: [w396 w405] -> w352
          tunnel: [w397 w404] -> w351
          tunnel: [w391 w400] -> w350
          tunnel: w354 -> [w395 w403]
          tunnel: [w390 w398] -> w359
          tunnel: w360 -> [w390 w398]
          frame False {
            n122 = Or(x=w394, y=w395) -> (x .or. y?=w393:bool)
            n123 = call "error_check_shutdown_freq_sweep.vi"(8:State."Sweeping down", "Boolean"=w393) -> (3:w391:T2)  [unwired: 9 in]
          }
          frame True {
            n124 = Or(x=w402, y=w403) -> (x .or. y?=w401:bool)
            n125 = call "error_check_shutdown_freq_sweep.vi"(8:State."Sweeping down", "Boolean"=w401) -> (3:w400:T2)  [unwired: 9 in]
          }
        }
      }
      frame "Sweeping down" {
        n126 = control-ref of="Status"() -> (w418:refnum<vi>)
        n127 = call "change_status.vi"("error in (no error)"=w428, "String"="Sweeping down the H field to zero...", "String in"=w418) -> ("error out"=w430:errorcluster)  [unwired: 8 in]
        n128 = call "disable.vi"("error in (no error)"=w430, "Array"=w423) -> ("error out"=w409:errorcluster)  [unwired: 9 in]
        n129 = call "disable.vi"("error in (no error)"=w409, "Array"=w424) -> ("error out"=w429:errorcluster)  [unwired: 9 in]
        n130 = call "disable.vi"("error in (no error)"=w429, "Array"=w425) -> ("error out"=w408:errorcluster)  [unwired: 9 in]
        n131 = call "disable.vi"("error in (no error)"=w408, "Array"=w407) -> ("error out"=w406:errorcluster)  [unwired: 9 in]
        n132 = call-poly <vilib>:"DAQmx Write.vi"("task/channels in"=w426, "data"=0.0, "error in"=w406) -> ("task out"=w415:refnum<k21>, "error out"=w413:errorcluster)  [unwired: 10 in, 1 out]
        n133 = Wait (ms)(milliseconds to wait=u32 1000) -> ()  [unwired: 1 out]
        n134 = call <vilib>:"DAQmx Stop Task.vi"("task/channels in"=w415, "error in"=w413) -> ("task out"=w414:refnum<k21>, "error out"=w412:errorcluster)  [unwired: 12 in]
        n135 = Or(x=w412, y=w421) -> (x .or. y?=w422:bool)
        n136 = call "error_check_shutdown_freq_sweep.vi"(8:State."Idle", "Boolean"=w422) -> (3:w420:T2)  [unwired: 9 in]
      }
      frame "Shutdown" {
        w436 = T3 3 items=["no dialog", "OK message", "continue or stop message", "OK message + warnings", "continue/stop + warnings"] ("type of dialog (OK msg:1)")
        n137 = control-ref of="Status"() -> (w458:refnum<vi>)
        n138 = call "change_status.vi"("error in (no error)"=w457, "String"="Shutting down...Sweeping field to zero...", "String in"=w458) -> ("error out"=w463:errorcluster)  [unwired: 8 in]
        n139 = call "disable.vi"("error in (no error)"=w463, "Array"=w461) -> ("error out"=w443:errorcluster)  [unwired: 9 in]
        n140 = call "disable.vi"("error in (no error)"=w443, "Array"=w460) -> ("error out"=w464:errorcluster)  [unwired: 9 in]
        n141 = call "disable.vi"("error in (no error)"=w464, "Array"=w459) -> ("error out"=w442:errorcluster)  [unwired: 9 in]
        n142 = call "disable.vi"("error in (no error)"=w442, "Array"=w440) -> ("error out"=w441:errorcluster)  [unwired: 9 in]
        n143 = call-poly <vilib>:"DAQmx Write.vi"("task/channels in"=w450, "data"=0.0, "error in"=w441) -> ("task out"=w448:refnum<k21>, "error out"=w449:errorcluster)  [unwired: 10 in, 1 out]
        n144 = Wait (ms)(milliseconds to wait=u32 1000) -> ()  [unwired: 1 out]
        n145 = call <vilib>:"DAQmx Stop Task.vi"("task/channels in"=w448, "error in"=w449) -> ("task out"=w453:refnum<k21>, "error out"=w455:errorcluster)  [unwired: 12 in]
        n146 = call <vilib>:"DAQmx Clear Task.vi"("task in"=w453, "error in"=w455) -> ("error out"=w446:errorcluster)  [unwired: 13 in]
        n147 = call <instrlib>:"niVNA Abort.vi"("instrument handle"=w447, "error in"=w446) -> ("instrument handle out"=w454:refnum<k15>, "error out"=w456:errorcluster)  [unwired: 12 in]
        n148 = call <instrlib>:"niVNA Close.vi"("instrument handle"=w454, "error in"=w456) -> ("error out"=w434:errorcluster)  [unwired: 13 in]
        n149 = property on="SpectrumGraph" class="XYGraph (strict)"(error in=w434, "Value"=cluster{"Field":dbl[], "Signal":dbl[]} {"Field"=[], "Signal"=[]} ("SpectrumGraph")) -> (error out=w433:errorcluster)  [unwired: 1 in, 1 out]
        n150 = control-ref of="Status"() -> (w439:refnum<vi>)
        n151 = call "change_status.vi"("error in (no error)"=w433, "String"="Off", "String in"=w439) -> ("error out"=w437:errorcluster)  [unwired: 8 in]
        n152 = call <vilib>:"Simple Error Handler.vi"("type of dialog (OK msg:1)"=w436, "error in (no error)"=w437) -> ("error out"=w435:errorcluster)  [unwired: 3 in, 4 out]
      }
    }
    n153 = event shown="[1] \"SpectrumGraph\": Mouse Down" {
      selector: _ -> [_ _ _]
      dyn-events: _ -> [_ _ _]
      timeout: 1 -> [_ _ _]
      event Timeout {
        n154 = event-data() -> ()  [unwired: 1 in, 3 out]
      }
      event "SpectrumGraph": Mouse Down {
        n155 = event-data() -> ("CtlRef"=w63:refnum<vi>, "Coords"=w64:T4)  [unwired: 1 in]
        n156 = invoke on="Invoke Node" class="XYGraph (strict)" method="Map Coords To XY"(reference=w63, "Coords"=w64) -> ("Map Coords To XY"=w65:bool, "XY"=w66:cluster{"X":dbl, "Y":dbl})  [unwired: 5 in, 5 out]
        n157 = case shown="True" w65 {
          tunnel: w66 -> [_ w67]
          frame False {
          }
          frame True {
            n158 = property on="Cursor" class="Clust (strict)"("Value"=w67) -> ()  [unwired: 2 in, 2 out]
          }
        }
      }
      event "Save Button": Value Change {
        n159 = event-data() -> ()  [unwired: 1 in, 1 out]
        n160 = property on="SpectrumGraph" class="XYGraph (strict)"() -> ("Value"=w68:cluster{"Field":dbl[], "Signal":dbl[]})  [unwired: 2 in, 2 out]
        n161 = Unbundle By Name(w68) -> ("Field"=w70:dbl[], "Signal"=w69:dbl[])
        n162 = call "Convert to Dynamic Data"("Array"=w70) -> ("Dynamic Data Type"=w73:dynamicdata)  [unwired: 3 in]
        n163 = call "Convert to Dynamic Data2"("Array"=w69) -> ("Dynamic Data Type"=w71:dynamicdata)  [unwired: 3 in]
        n164 = Merge Signals(w73, w71) -> (w72:dynamicdata)
        n165 = call "Write To Measurement File"("Signals"=w72) -> ()  [unwired: 16 in, 3 out]
      }
    }
  }
  "Error Out" <- w14
  "VNA Name Out" <- w13
  "DAQ channel Out" <- w12
  "Cursor" <- cluster{"x":dbl, "y":dbl} {"x"=0.0, "y"=0.0} ("Cursor")
